vi "SetDarConvIntercept.vi"(8 "error in (no error)":errorcluster, 10 "dparConvIntercept":dbl, 11 "dvotAFTKinetics in":refnum<class "dvotAFTKinetics.lvclass">) -> (0 "error out":errorcluster, 3 "dvotAFTKinetics out":refnum<class "dvotAFTKinetics.lvclass">)   [LabVIEW 2012, in "dvotAFTKinetics.lvclass"]
uses:
  dvotAFTKinetics.lvclass
  dvotAFTKinetics.lvclass/dvotAFTKinetics.ctl
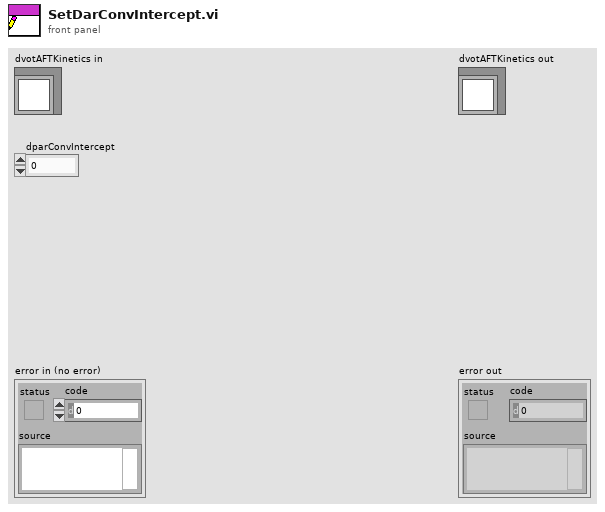
[diagram p1: front panel]
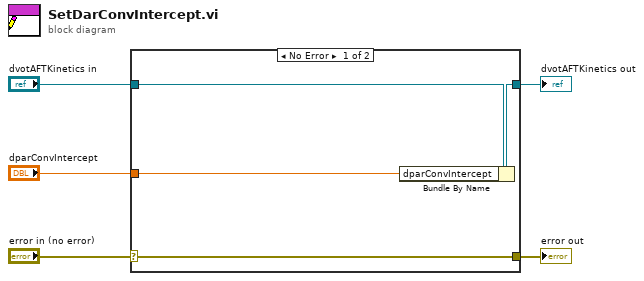
[diagram p0: block diagram]
diagram:
  n1 = case shown="No Error" "error in (no error)" {
    selector: "error in (no error)" -> [w9 w10]
    tunnel: [w9 w10] -> w4
    tunnel: [w7 w11] -> w2
    tunnel: "dvotAFTKinetics in" -> [w8 w11]
    tunnel: "dparConvIntercept" -> [w6 _]
    frame No Error {
      n2 = Bundle By Name(cluster=w8, "dparConvIntercept"=w6) -> (w7:refnum<class "dvotAFTKinetics.lvclass">)
    }
    frame Error {
    }
  }
  "error out" <- w4
  "dvotAFTKinetics out" <- w2
